vi "Q_learning_update_env.vi"(8 "step_counter":dbl, 9 "episode":dbl, 11 "S":string) -> (2 "Print":string)   [LabVIEW 2010]
uses:
  Q_learning_Global.vi
panel:
  out "env_list":string
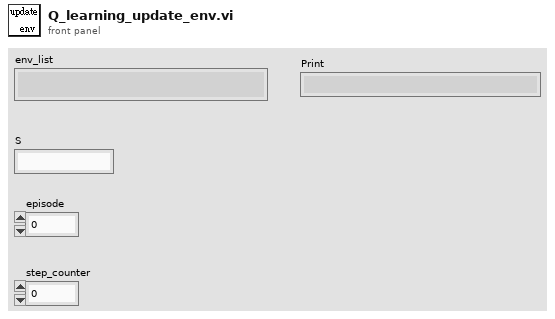
[diagram p1: front panel]
types:
  T1 = cluster{"N_STATES":dbl, "EPSILON":dbl, "ALPHA":dbl, "GAMMA":dbl, "MAX_EPISODES":dbl, "FRESH_TIME":dbl, "ACTIONS":string[]}
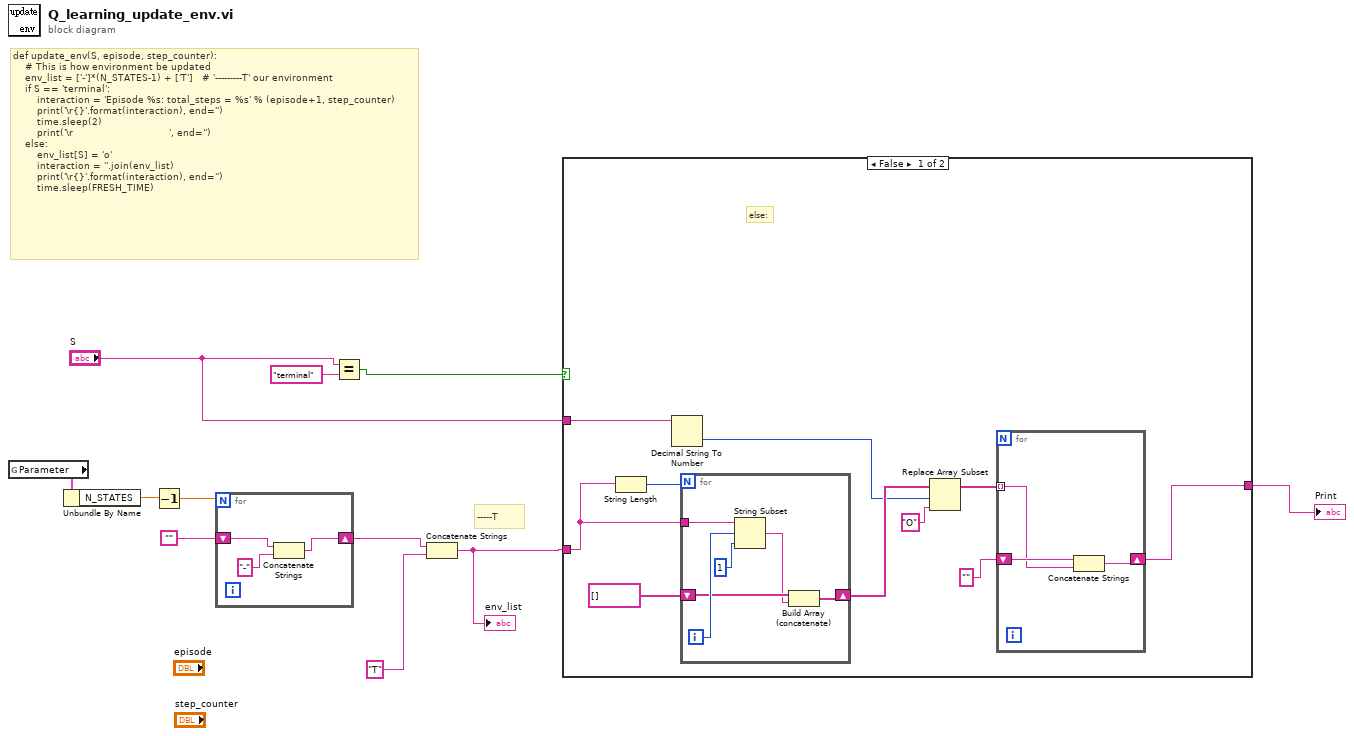
[diagram p0: block diagram]
diagram:
  # "-----T"
  # "def update_env(S, episode, step_counter):\n    # This is how environment be updated\n    env_list = ['-']*(N_STATES-1) + ['T']   # '---------T' our environment\n    if S == 'terminal':\n        interaction = 'Episode %s: total_steps = %s' % (episode+1, step_counter)\n        print('\\r{}'.format(interaction), end='')\n        time.sleep(2)\n        print('\\r                                ', end='')\n    else:\n        env_list[S] = 'o'\n        interaction = ''.join(env_list)\n        print('\\r{}'.format(interaction), end='')\n        time.sleep(FRESH_TIME)"
  n1 = global read "Q_learning_Global.vi" "Parameter"() -> (w11:T1)
  n2 = Unbundle By Name(w11) -> ("N_STATES"=w10:dbl)
  n3 = Decrement(x=w10) -> (x-1=w9:dbl)
  n4 = for {
    N: w9 -> [_]
    shift-right: [w12] -> w7
    shift-left: "" -> [w14]
    n5 = Concatenate Strings(w14, "-") -> (w12:string)
  }
  n6 = Equal?(x="S", y="terminal") -> (x = y?=w4:bool)
  n7 = Concatenate Strings(w7, "T") -> (w2:string)
  "env_list" <- w2
  n8 = case shown="False" w4 {
    tunnel: "S" -> [w24 _]
    tunnel: w2 -> [w22 _]
    tunnel: [w15 _] -> w1
    frame False {
      # "else:"
      n9 = String Length(string=w22) -> (length=w23:i32)
      n10 = Decimal String To Number(string=w24) -> (number=w19:i32)  [unwired: 2 in, 1 out]
      n11 = for {
        N: w23 -> [_]
        tunnel: w22 -> [w33]
        shift-right: [w30] -> w20
        shift-left: string[] [] -> [w31]
        i -> [w32]
        n12 = String Subset(string=w33, offset (0)=w32, length (rest)=1 ("length (rest)")) -> (substring=w29:string)
        n13 = Build Array (concatenate)(w31, w29) -> (w30:string[])
      }
      n14 = Replace Array Subset(array=w20, new element="O" ("new element/subarray"), index=w19) -> (w17:string[])
      n15 = for {
        tunnel: w17 -> [w25] mode=indexing
        shift-right: [w26] -> w15
        shift-left: "" -> [w27]
        n16 = Concatenate Strings(w27, w25) -> (w26:string)
      }
    }
    frame True {
    }
  }
  "Print" <- w1
